vi "ROI entry-Event handler-Equal Size.vi"   [LabVIEW 2017]
uses:
  ROI Entry screen/Globals/gl_ROI Entry UI globals.vi
types:
  T1 = typedef "ROI entry screen ctrl refs cluster.ctl" = cluster{"Done button":refnum<vi>, "Imaging button":refnum<vi>, "Acquisition button":refnum<vi>, "POI dwell time (us)":refnum<vi>, "Scan dwell time per pixel (us)":refnum<vi>, "# of planes":refnum<vi>, "Zoom Ctrl":refnum<vi>, "Equal size":refnum<vi>, "Channel":refnum<vi>, "Image Display":refnum<vi>, "Z-Plane Selector":refnum<vi>, "Number of lines left":refnum<vi>, "Z-stack folder path":refnum<vi>, "POI Density":refnum<vi>, "Arb Plane Entry":refnum<vi>, "Whole plane":refnum<vi>, "Clear Last":refnum<vi>, "Clear All":refnum<vi>, "Trial Length (sec)":refnum<vi>, "Palette Type":refnum<vi>, "Intensity slider":refnum<vi>, "# POI":refnum<vi>, "Max Z Proj":refnum<vi>, "Zplane ind":refnum<vi>, "Wavelength (nm)":refnum<vi>, "Number of Trials":refnum<vi>, "Funct stim.trig.enable":refnum<vi>, "Funct stim.trig.delay (s)":refnum<vi>, "Line Mode":refnum<vi>, "Step size (µm)":refnum<vi>, "ROI move mode":refnum<vi>, "Cool-down time (s)":refnum<vi>, "Enable cool-down time":refnum<vi>, "Motor Z ind. (um)":refnum<vi>, "AOL Z ind. (um)":refnum<vi>, "Load Reference Image":refnum<vi>}
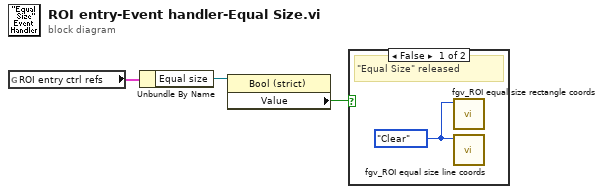
[diagram p0: block diagram]
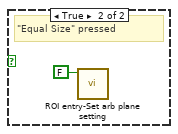
[diagram p2: hidden frame]
diagram:
  n1 = global read "gl_ROI Entry UI globals.vi" "ROI entry ctrl refs"() -> (w2:T1)
  n2 = Unbundle By Name(w2) -> ("Equal size"=w3:refnum<vi>)
  n3 = property on="Property Node" class="Bool (strict)"(reference=w3) -> ("Value"=w1:bool)  [unwired: 1 in, 2 out]
  n4 = case shown="False" w1 {
    frame False {
      w4 = enum16{"Intialize", "Write", "Read", "Clear"}."Clear" ("Function")
      # "\"Equal Size\" released"
      n5 = call "fgv_ROI equal size rectangle coords.vi"("Function"=w4) -> ()  [unwired: 9 in, 2 out]
      n6 = call "fgv_ROI equal size line coords.vi"("Function"=w4) -> ()  [unwired: 9 in, 2 out]
    }
    frame True {
      # "\"Equal Size\" pressed"
      n7 = call "ROI entry-Set arb plane setting.vi"("\"Arb plane entry\" button's value"=FALSE ("\"Arb plane entry\" button's value")) -> ()  [unwired: 10 in, 1 out]
    }
  }
